vi "Configure Active DUT Airplane Mode Enabled.vi"(8 "error in (no error)":errorcluster, 10 "Airplane Mode (Off)":bool, 11 "VISA resource name":refnum<visa-resource-name>) -> (0 "error out":errorcluster, 3 "VISA resource name out":refnum<visa-resource-name>)   [LabVIEW 2020, in "Rohde&Schwarz CMXP Base.lvlib"]
doc: "Switches the airplane mode at the DUT on or off.\n\nAttribute:\nRSCMXPBASE_ATTR_ACTIVE_DUT_AIRPLANE_MODE_ENABLED\n\nRemote-control command:\nPROCedure:DUT:CONTrol:AIRPlane"
uses:
  <instrlib>/Rohde&Schwarz CMXP Base/Rohde&Schwarz CMXP Base.lvlib
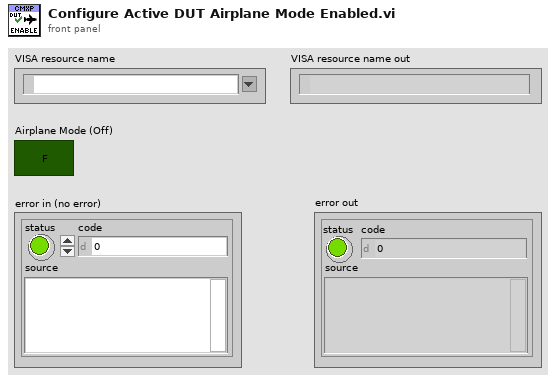
[diagram p1: front panel]
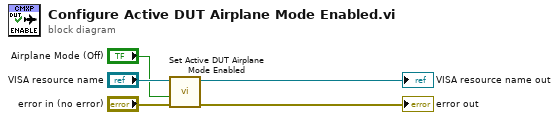
[diagram p0: block diagram]
diagram:
  n1 = call "Set Active DUT Airplane Mode Enabled"("error in (no error)"="error in (no error)", "Active DUT Airplane Mode Enabled (OFF)"="Airplane Mode (Off)", "instrument handle"="VISA resource name") -> ("error out"=→"error out":errorcluster, "instrument handle out"=→"VISA resource name out":refnum<visa-resource-name>)  [unwired: 7 in]
